vi "Manage Settings.vi"(2 "error in (no error)":errorcluster, 3 "Config Cluster Array Input":T1[](array[typedef]), 4 "Save Current Values":bool) -> (0 "error out":errorcluster, 1 "file path":path)   [LabVIEW 2020, in "Settings Manager.lvlib"]
uses:
  Type Defs/Config Type Cluster.ctl
  <vilib>/Utility/config.llb/Write Key (String).vi
  <vilib>/Utility/config.llb/Read Key (String).vi
  <vilib>/Utility/config.llb/Read Key (U32).vi
  <vilib>/Utility/config.llb/Read Key (Double).vi
  <vilib>/Utility/config.llb/Read Key (Path).vi
  <vilib>/Utility/config.llb/Read Key (Boolean).vi
  Settings Manager.lvlib
  <vilib>/Utility/config.llb/NI_LVConfig.lvlib
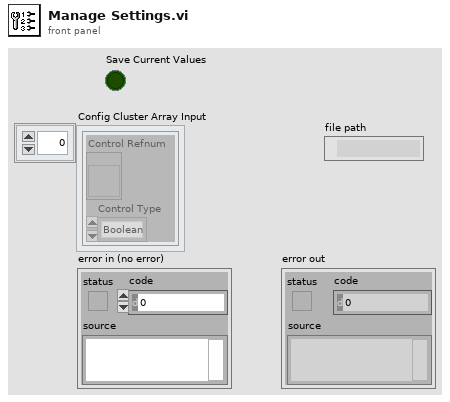
[diagram p1: front panel]
types:
  T1 = typedef "Settings Manager.lvlib/Config Type Cluster.ctl" = cluster{"Control Refnum":refnum<vi>, "Control Type":enum16{"Boolean", "String", "Integer", "Float", "Path"}}
  T2 = typedef "NI_LVConfig.lvlib/Config Data RefNum.ctl" = refnum<k1>
  T3 = enum16{"Boolean", "String", "Integer", "Float", "Path"}
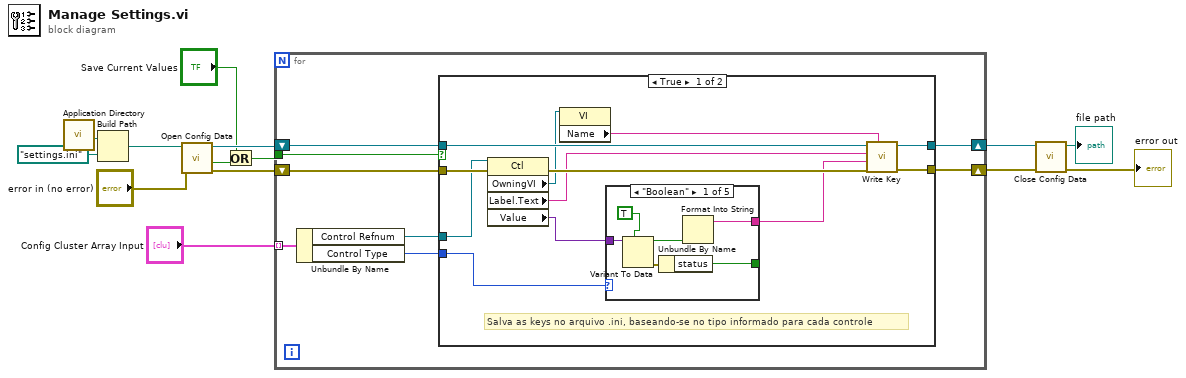
[diagram p0: block diagram]
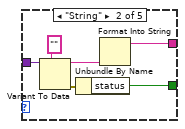
[diagram p2: hidden frame]
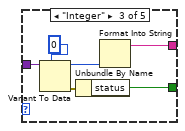
[diagram p3: hidden frame]
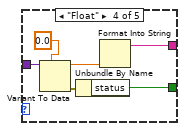
[diagram p4: hidden frame]
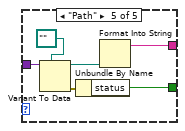
[diagram p5: hidden frame]
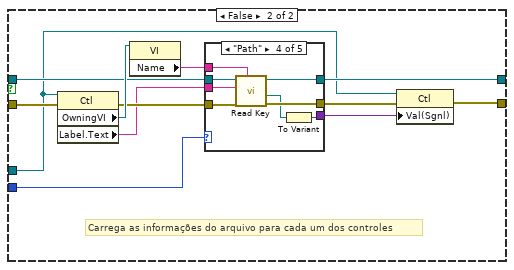
[diagram p6: hidden frame]
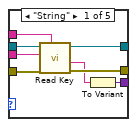
[diagram p7: hidden frame]
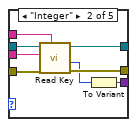
[diagram p8: hidden frame]
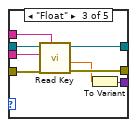
[diagram p9: hidden frame]
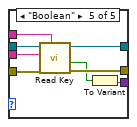
[diagram p10: hidden frame]
diagram:
  n1 = call <vilib>:"Application Directory.vi"() -> ("Application Directory"=w14:path)
  n2 = Build Path(base path=w14, name or relative path=path "settings.ini") -> (appended path=w12:path)
  n3 = call <vilib>:"Open Config Data.vi"("error in (no error)"="error in (no error)", "configuration file path"=w12) -> ("error out"=w10:errorcluster, "file created?"=w2:bool, "refnum"=w11:T2)  [unwired: 7 in]
  n4 = Or(x="Save Current Values", y=w2) -> (x .or. y?=w3:bool)
  n5 = for {
    tunnel: "Config Cluster Array Input" -> [w18] mode=indexing
    shift-right: [w19] -> w8
    shift-left: w10 -> [w22]
    shift-right: [w20] -> w9
    shift-left: w11 -> [w21]
    tunnel: w3 -> [w15]
    n6 = Unbundle By Name(w18) -> ("Control Refnum"=w17:refnum<vi>, "Control Type"=w16:T3)
    n7 = case shown="True" w15 {
      tunnel: w22 -> [w34 w76]
      tunnel: w21 -> [w32 w74]
      tunnel: [w30 w73] -> w20
      tunnel: [w29 w68] -> w19
      tunnel: w17 -> [w24 w67]
      tunnel: w16 -> [w23 w65]
      frame True {
        # "Salva as keys no arquivo .ini, baseando-se no tipo informado para cada controle"
        n8 = property class="Ctl"(reference=w24, error in=w34) -> (error out=w33:errorcluster, "OwningVI"=w28:refnum<vi>, "Label.Text"=w31:string, "Value"=w26:variant)  [unwired: 1 out]
        n9 = property class="VI"(reference=w28) -> ("Name"=w27:string)  [unwired: 1 in, 2 out]
        n10 = case shown="\"Boolean\"" w23 {
          tunnel: [w38 w44 w50 w56 w62] -> _
          tunnel: w26 -> [w40 w46 w52 w58 w64]
          tunnel: [w36 w42 w48 w54 w60] -> w25
          frame "Boolean" {
            n11 = Variant To Data(type=TRUE, Variant=w40) -> (data=w37:bool, error out=w39:errorcluster)  [unwired: 1 in]
            n12 = Unbundle By Name(w39) -> ("status"=w38:bool)
            n13 = Format Into String(w37) -> (resulting string=w36:string)  [unwired: 3 in, 1 out]
          }
          frame "String" {
            n14 = Variant To Data(type="", Variant=w46) -> (data=w43:string, error out=w45:errorcluster)  [unwired: 1 in]
            n15 = Unbundle By Name(w45) -> ("status"=w44:bool)
            n16 = Format Into String(w43) -> (resulting string=w42:string)  [unwired: 3 in, 1 out]
          }
          frame "Integer" {
            n17 = Variant To Data(type=0, Variant=w52) -> (data=w49:i32, error out=w51:errorcluster)  [unwired: 1 in]
            n18 = Unbundle By Name(w51) -> ("status"=w50:bool)
            n19 = Format Into String(w49) -> (resulting string=w48:string)  [unwired: 3 in, 1 out]
          }
          frame "Float" {
            n20 = Variant To Data(type=0.0, Variant=w58) -> (data=w55:dbl, error out=w57:errorcluster)  [unwired: 1 in]
            n21 = Unbundle By Name(w57) -> ("status"=w56:bool)
            n22 = Format Into String(w55) -> (resulting string=w54:string)  [unwired: 3 in, 1 out]
          }
          frame "Path" {
            n23 = Variant To Data(type=path "", Variant=w64) -> (data=w61:path, error out=w63:errorcluster)  [unwired: 1 in]
            n24 = Unbundle By Name(w63) -> ("status"=w62:bool)
            n25 = Format Into String(w61) -> (resulting string=w60:string)  [unwired: 3 in, 1 out]
          }
        }
        n26 = call-poly <vilib>:"Write Key.vi"("section"=w27, "error in (no error)"=w33, "value"=w25, "key"=w31, "refnum"=w32) -> ("error out"=w29:errorcluster, "refnum out"=w30:T2)  [unwired: 4 in, 1 out]
      }
      frame False {
        # "Carrega as informações do arquivo para cada um dos controles"
        n27 = property class="Ctl"(reference=w67, error in=w76) -> (error out=w72:errorcluster, "OwningVI"=w75:refnum<vi>, "Label.Text"=w71:string)  [unwired: 1 out]
        n28 = property class="VI"(reference=w75) -> ("Name"=w70:string)  [unwired: 1 in, 2 out]
        n29 = case shown="\"Path\"" w65 {
          tunnel: w74 -> [w84 w92 w100 w108 w116]
          tunnel: [w83 w91 w99 w107 w115] -> w73
          tunnel: w72 -> [w82 w90 w98 w106 w114]
          tunnel: w71 -> [w81 w89 w97 w105 w113]
          tunnel: w70 -> [w80 w88 w96 w104 w112]
          tunnel: [w79 w87 w95 w103 w111] -> w69
          tunnel: [w77 w85 w93 w101 w110] -> w66
          frame "String" {
            n30 = call-poly <vilib>:"Read Key.vi"("section"=w80, "error in (no error)"=w82, "key"=w81, "refnum"=w84) -> ("error out"=w79:errorcluster, "value"=w78:string, "refnum out"=w83:T2)  [unwired: 4 in, 1 out]
            n31 = To Variant(anything=w78) -> (Variant=w77:variant)
          }
          frame "Integer" {
            n32 = call-poly <vilib>:"Read Key.vi"("section"=w88, "error in (no error)"=w90, "key"=w89, "refnum"=w92) -> ("error out"=w87:errorcluster, "value"=w86:u32, "refnum out"=w91:T2)  [unwired: 4 in, 1 out]
            n33 = To Variant(anything=w86) -> (Variant=w85:variant)
          }
          frame "Float" {
            n34 = call-poly <vilib>:"Read Key.vi"("section"=w96, "error in (no error)"=w98, "key"=w97, "refnum"=w100) -> ("error out"=w95:errorcluster, "value"=w94:dbl, "refnum out"=w99:T2)  [unwired: 4 in, 1 out]
            n35 = To Variant(anything=w94) -> (Variant=w93:variant)
          }
          frame "Path" {
            n36 = call-poly <vilib>:"Read Key.vi"("section"=w104, "error in (no error)"=w106, "key"=w105, "refnum"=w108) -> ("error out"=w103:errorcluster, "value"=w102:path, "refnum out"=w107:T2)  [unwired: 4 in, 1 out]
            n37 = To Variant(anything=w102) -> (Variant=w101:variant)
          }
          frame "Boolean" {
            n38 = call-poly <vilib>:"Read Key.vi"("section"=w112, "error in (no error)"=w114, "key"=w113, "refnum"=w116) -> ("error out"=w111:errorcluster, "value"=w109:bool, "refnum out"=w115:T2)  [unwired: 4 in, 1 out]
            n39 = To Variant(anything=w109) -> (Variant=w110:variant)
          }
        }
        n40 = property class="Ctl"(reference=w67, error in=w69, "Val(Sgnl)"=w66) -> (error out=w68:errorcluster)  [unwired: 1 out]
      }
    }
  }
  n41 = call <vilib>:"Close Config Data.vi"("error in (no error)"=w8, "refnum"=w9) -> ("error out"=→"error out":errorcluster, "file path"=→"file path":path)  [unwired: 8 in]
